vi "PipBoy_EnqueueIfEmpty.vi"(6 "timeout in ms (-1)":i32=-1, 8 "error in (no error)":errorcluster, 9 "Message Data":variant, 10 "Message":string="AcquirePipBoy", 11 "Message Queue":refnum<queue>) -> (0 "error out":errorcluster)   [LabVIEW 2014]
uses:
  modules/support/Message Queue/Message Cluster.ctl
  modules/support/Message Queue/Message Queue.lvlib
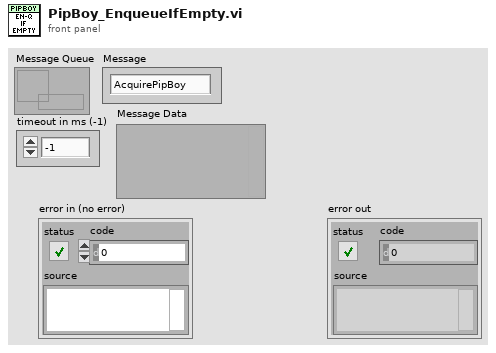
[diagram p1: front panel]
types:
  T1 = typedef "Message Queue.lvlib/Message Cluster.ctl" = cluster{"Message":string, "Message Data":variant}
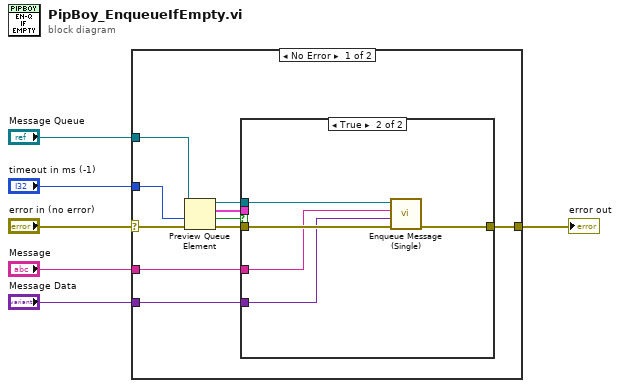
[diagram p0: block diagram]
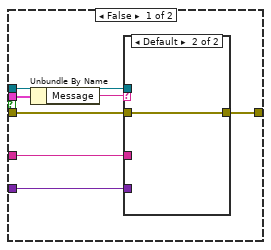
[diagram p2: hidden frame]
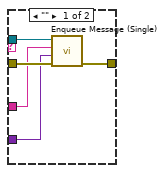
[diagram p3: hidden frame]
diagram:
  n1 = case shown="No Error" "error in (no error)" {
    selector: "error in (no error)" -> [w11 w35]
    tunnel: "timeout in ms (-1)" -> [w16 _]
    tunnel: "Message Queue" -> [w10 _]
    tunnel: [w12 w35] -> w4
    tunnel: "Message" -> [w9 _]
    tunnel: "Message Data" -> [w8 _]
    frame No Error {
      n2 = Preview Queue Element(queue=w10, timeout in ms (-1)=w16, error in (no error)=w11) -> (queue out=w13:refnum<queue>, element=w7:T1, timed out?=w15:bool, error out=w14:errorcluster)
      n3 = case shown="True" w15 {
        tunnel: w14 -> [w21 w34]
        tunnel: w13 -> [w19 w33]
        tunnel: [w20 w32] -> w12
        tunnel: w9 -> [w18 w31]
        tunnel: w8 -> [w17 w30]
        tunnel: w7 -> [w23 _]
        frame False {
          n4 = Unbundle By Name(w23) -> ("Message"=w22:string)
          n5 = case shown="Default" w22 {
            tunnel: w21 -> [w28 w29]
            tunnel: [w27 w29] -> w20
            tunnel: w19 -> [w26 _]
            tunnel: w18 -> [w25 _]
            tunnel: w17 -> [w24 _]
            frame "" {
              n6 = call "Enqueue Message (Single).vi"("error in (no error)"=w28, "Message Data"=w24, "Message"=w25, "Message Queue"=w26) -> ("error out"=w27:errorcluster)  [unwired: 6 in, 1 out]
            }
            frame Default {
            }
          }
        }
        frame True {
          n7 = call "Enqueue Message (Single).vi"("error in (no error)"=w34, "Message Data"=w30, "Message"=w31, "Message Queue"=w33) -> ("error out"=w32:errorcluster)  [unwired: 6 in, 1 out]
        }
      }
    }
    frame Error {
    }
  }
  "error out" <- w4
